vi "SeparateRecords.vi"(8 "error in (no error)":errorcluster, 11 "ParseGDSII in":refnum<class "ParseGDSII.lvclass">) -> (0 "error out":errorcluster, 3 "ParseGDSII out":refnum<class "ParseGDSII.lvclass">)   [LabVIEW 2020, in "ParseGDSII.lvclass"]
uses:
  ParseGDSII.lvclass
  ParseGDSII.lvclass/ParseGDSII.ctl
panel:
  out "Record Array":string[](array[string])
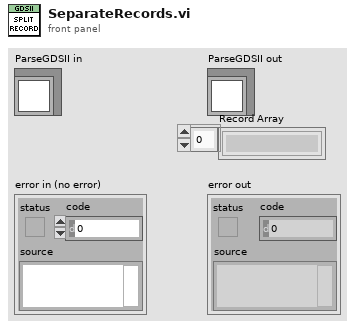
[diagram p1: front panel]
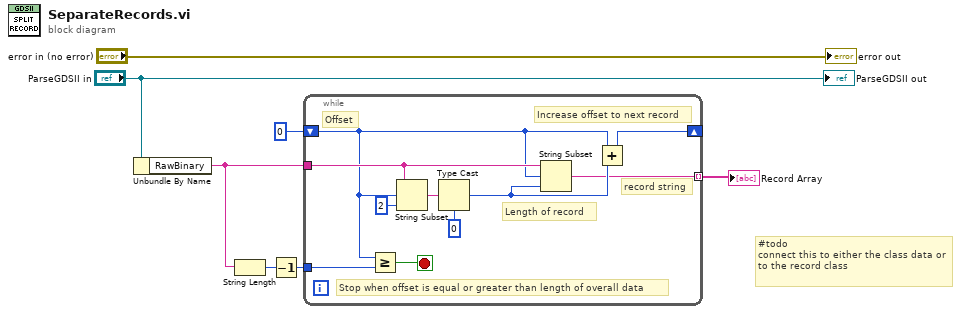
[diagram p0: block diagram]
diagram:
  # "#todo\nconnect this to either the class data or to the record class"
  n1 = Unbundle By Name("ParseGDSII in") -> ("RawBinary"=w4:string)
  n2 = String Length(string=w4) -> (length=w6:i32)
  n3 = Decrement(x=w6) -> (x-1=w5:i32)
  n4 = while {
    tunnel: w5 -> [w17]
    tunnel: w4 -> [w12]
    shift-right: [w10] -> _
    shift-left: 0 -> [w11]
    tunnel: [w8] -> w1 mode=indexing
    stop <- w16 stop-if-true
    # "record string"
    # "Stop when offset is equal or greater than length of overall data"
    # "Increase offset to next record"
    # "Length of record"
    # "Offset"
    n5 = Greater Or Equal?(x=w11, y=w17) -> (x >= y?=w16:bool)
    n6 = String Subset(string=w12, offset (0)=w11, length (rest)=2 ("length (rest)")) -> (substring=w14:string)
    n7 = Type Cast(type=i16 0, x=w14) -> (*(type *) &x=w9:i16)
    n8 = String Subset(string=w12, offset (0)=w11, length (rest)=w9) -> (substring=w8:string)
    n9 = Add(x=w11, y=w9) -> (x+y=w10:i32)
  }
  "Record Array" <- w1
  "error out" <- "error in (no error)"
  "ParseGDSII out" <- "ParseGDSII in"
